vi "Christinas Flow Control Program.vi"() -> ()   [LabVIEW 2015]
uses:
  Alicat Device.lvclass
  Reusable/Session APIs/File Access/Config Data/Config Session.ctl
  Reusable/Session APIs/File Access/Config Data/Config Data.lvclass
  Reusable/Session APIs/Serial/Serial Session.lvclass
  <userlib>/_Session Fwk/Typedefs/Session Handle.ctl
  <userlib>/_Session Fwk/Session - Root.lvclass
  Reusable/Session Log/System Log.lvclass
  Reusable/Session Log/System Log.lvclass/System Log.ctl
  Reusable/Session APIs/File Access/Config Data/Config Data.lvclass/Config Data.ctl
  Reusable/Session APIs/Text Communication/Text Device Session.lvclass/Text Device Session.ctl
  Configurable Device/Configurable Device.lvclass/Configurable Device.ctl
  Alicat Device.lvclass/Alicat Device.ctl
  Data/Alicat Data.lvclass
  Reusable/Session APIs/Text Communication/Write hSysLog.vi
  Configurable Device/Write Handle.vi
  Accessors/Write ID.vi
  Accessors/Write Session Handle.vi
  Accessors/Read Type.vi
  Reusable/Session Log/Accessors/Write Main Path.vi
  Reusable/Session APIs/File Access/Config Data/Accessors/Write Cfg Path.vi
  Reusable/Data/Read measTime.vi
  Reusable/Data/Data.lvclass
panel:
  in  "Limonene SP":dbl
  in  "Nitrogen SP":dbl
  in  "Ozone SP":dbl
  out "error out":errorcluster
  out "Acquisition Time":timestamp format="%<%H:%M:%S%2u>T"
  out "Limonene":T1
  out "Nitrogen":T1
  out "Ozone":T1
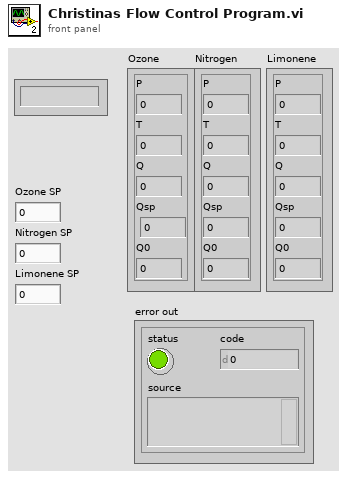
[diagram p1: front panel]
types:
  T1 = cluster{"P":dbl, "T":dbl, "Q":dbl, "Qsp":dbl, "Q0":dbl}
  T2 = typedef "Session - Root.lvclass/Session Handle.ctl" = refnum<data-value>
  T3 = typedef "Config Data.lvclass/Config Session.ctl" = refnum<data-value>
  T4 = cluster{"Accessors:Data[0]":sgl, "Accessors:Data[1]":sgl, "Accessors:Data[2]":sgl, "Accessors:Data[3]":sgl, "Accessors:Data[4]":sgl}
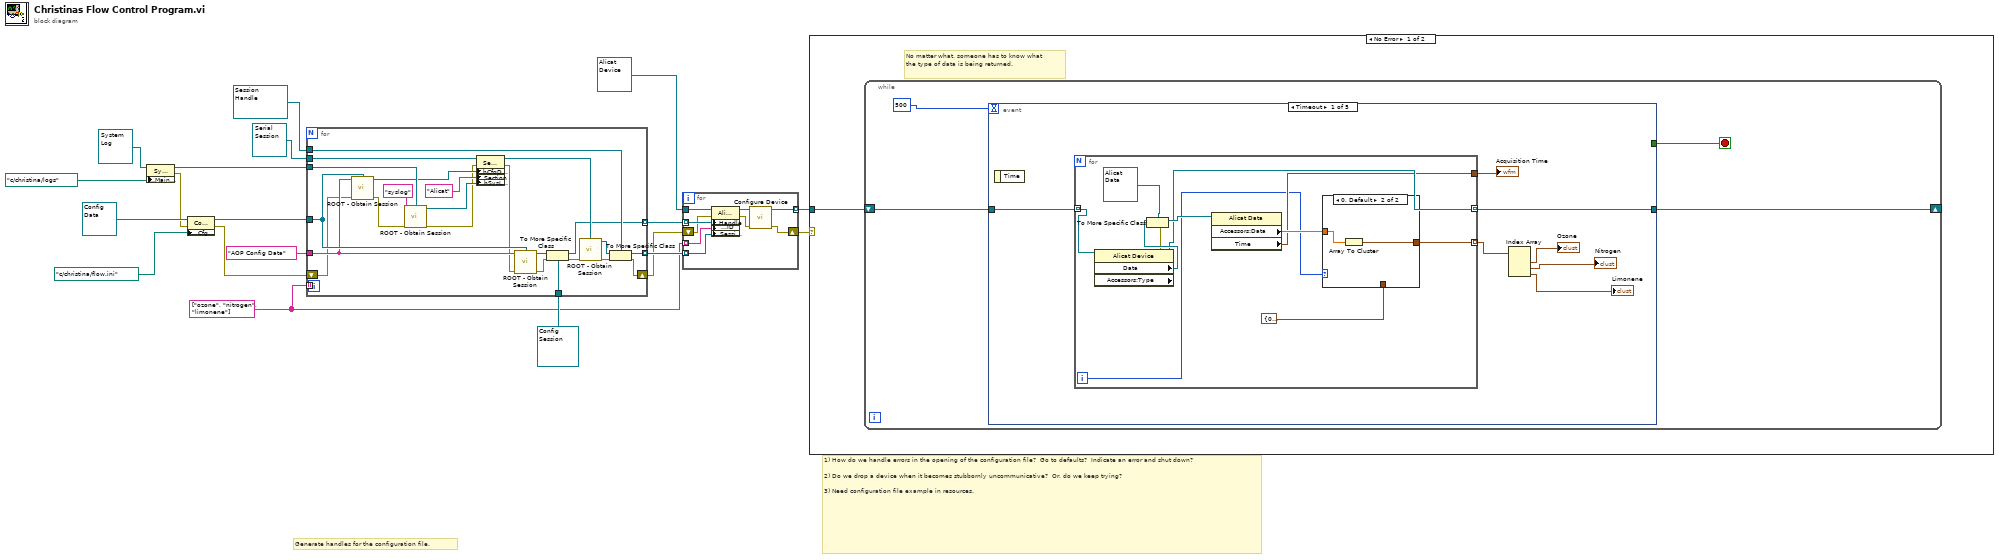
[diagram p0: block diagram]
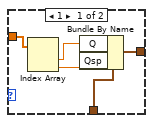
[diagram p2: hidden frame]
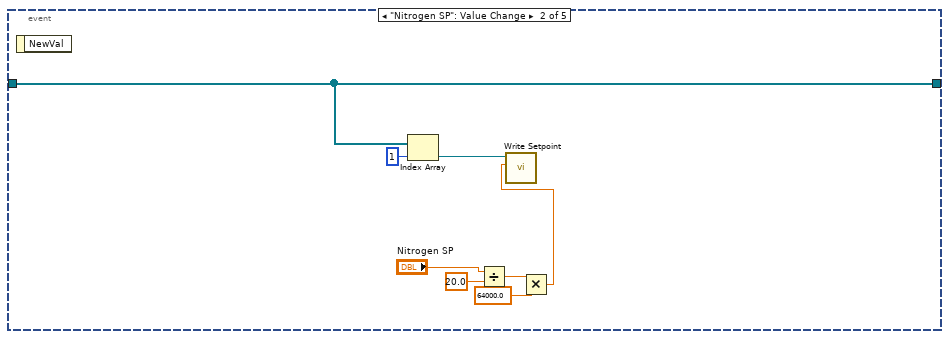
[diagram p3: hidden frame]
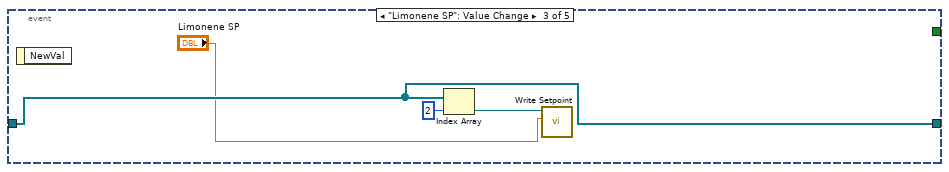
[diagram p4: hidden frame]
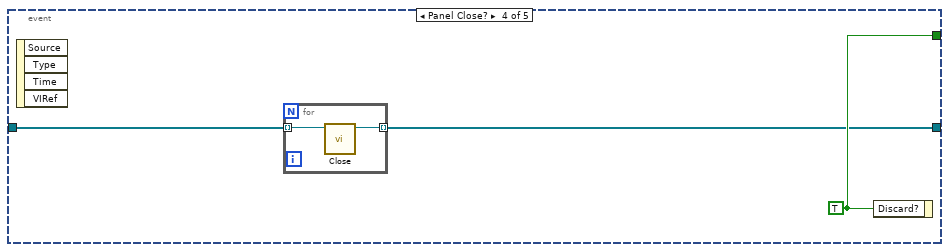
[diagram p5: hidden frame]
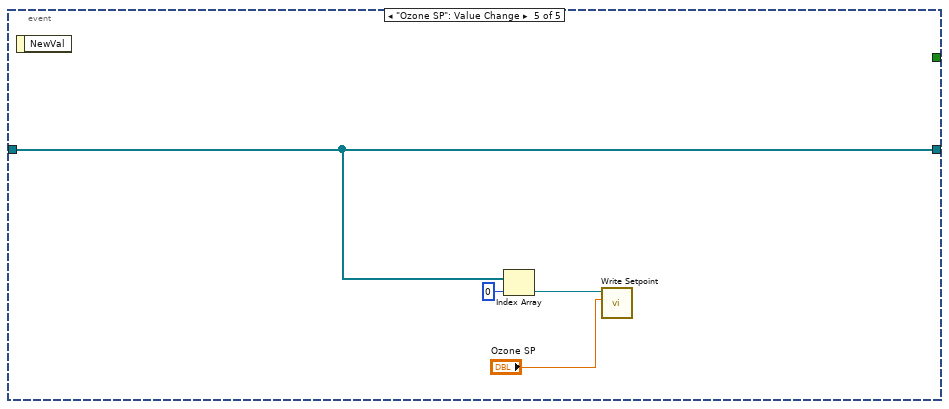
[diagram p6: hidden frame]
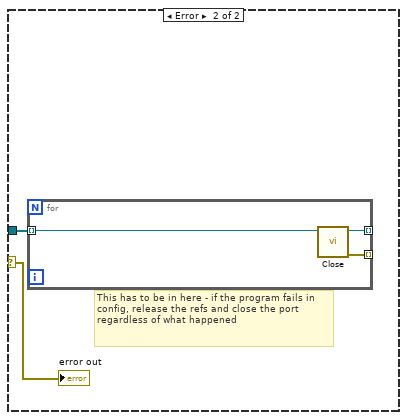
[diagram p7: hidden frame]
diagram:
  w2 = string[] ["ozone", "nitrogen", "limonene"] ("Array")
  # "1) How do we handle errors in the opening of the configuration file?  Go to defaults?  Indicate an error and shut down?\n\n2) Do we drop a device when it becomes stubbornly uncommunicative?  Or, do we keep trying?\n\n3) Need configuration file example in resources."
  # "Generate handles for the configuration file."
  n1 = property class="Sys Log"(reference=refnum<class "System Log.lvclass"> refnum ("Sys Log"), "Accessors:Main Path"=path "c:/christina/logs" ("Main Path")) -> (reference out=w9:refnum<class "System Log.lvclass">, error out=w4:errorcluster)  [unwired: 1 in]
  n2 = property class="Config Data"(reference=refnum<class "Config Data.lvclass"> refnum ("Config Data"), error in=w4, "Accessors:Cfg Path"=path "c:/christina/flow.ini" ("Path")) -> (reference out=w7:refnum<class "Config Data.lvclass">, error out=w3:errorcluster)
  n3 = for {
    tunnel: T3 refnum ("Session Handle") -> [w42]
    tunnel: [w28] -> w6 mode=indexing
    tunnel: "AOP Config Data" ("Session Name ()") -> [w26]
    tunnel: refnum<class "Serial Session.lvclass"> refnum ("Serial Session") -> [w40]
    tunnel: T2 refnum ("Session Handle") -> [w36]
    tunnel: [w35] -> w12 mode=indexing
    tunnel: w9 -> [w34]
    tunnel: w2 -> [_] mode=indexing
    tunnel: w7 -> [w27]
    shift-right: [w24] -> w1
    shift-left: w3 -> [w23]
    n4 = call <userlib>:"ROOT - Obtain Session.vi"("Session Name ()"=w26, "OBJ - Session"=w27, "error in (no error)"=w23) -> ("Session Handle"=w25:T2, "error out"=w22:errorcluster)  [unwired: 10 in, 1 out]
    n5 = call <userlib>:"ROOT - Obtain Session.vi"("Session Name ()"="syslog", "OBJ - Session"=w34, "error in (no error)"=w22) -> ("Session Handle"=w32:T2, "error out"=w21:errorcluster)  [unwired: 10 in, 1 out]
    n6 = property class="Serial Session"(reference=w40, error in=w21, "Accessors:hCfgData"=w25, "Accessors:Section"="Alicat" ("Section"), "Accessors:hSysLog"=w32) -> (reference out=w39:refnum<class "Serial Session.lvclass">, error out=w20:errorcluster)
    n7 = call <userlib>:"ROOT - Obtain Session.vi"("Session Name ()"=w26, "OBJ - Session"=w27, "error in (no error)"=w20) -> ("Session Handle"=w31:T2, "error out"=w41:errorcluster)  [unwired: 10 in, 1 out]
    n8 = To More Specific Class(target class=w42, reference=w31, error in=w41) -> (specific class reference=w28:T3, error out=w30:errorcluster)
    n9 = call <userlib>:"ROOT - Obtain Session.vi"("OBJ - Session"=w39, "error in (no error)"=w30) -> ("Session Handle"=w37:T2, "error out"=w29:errorcluster)  [unwired: 11 in, 1 out]
    n10 = To More Specific Class(target class=w36, reference=w37, error in=w29) -> (specific class reference=w35:T2, error out=w24:errorcluster)
  }
  n11 = for {
    tunnel: w2 -> [w50] mode=indexing
    tunnel: [w46] -> w18 mode=indexing
    tunnel: refnum<class "Alicat Device.lvclass"> refnum ("Alicat Device in") -> [w51]
    tunnel: w6 -> [w49] mode=indexing
    tunnel: w12 -> [w44] mode=indexing
    shift-right: [w45] -> w19
    shift-left: w1 -> [w43]
    n12 = property class="Alicat Device"(reference=w51, error in=w43, "Accessors:Handle"=w49, "Accessors:ID"=w50, "Accessors:Session Handle"=w44) -> (reference out=w47:refnum<class "Alicat Device.lvclass">, error out=w48:errorcluster)
    n13 = call-dynamic "Configure Device.vi"("error in"=w48, "Alicat Device in"=w47) -> ("error out"=w45:errorcluster, "Alicat Device out"=w46:refnum<class "Alicat Device.lvclass">)  [unwired: 8 in]
  }
  n14 = case shown="No Error" w19 {
    selector: w19 -> [_ w103]
    tunnel: w18 -> [w52 w104]
    frame No Error {
      # "No matter what, someone has to know what the type of data is being returned."
      n15 = while {
        shift-right: [w55] -> _
        shift-left: w52 -> [w56]
        stop <- w53 stop-if-true
        n16 = event shown="[0] Timeout" {
          selector: _ -> [_ _ _ _ _]
          dyn-events: _ -> [_ _ _ _ _]
          timeout: 500 -> [_ _ _ _ _]
          tunnel: w56 -> [w63 w89 w91 w95 w100]
          tunnel: [w62 w89 w91 w94 w100] -> w55
          tunnel: [_ _ _ w96 _] -> w53
          event Timeout {
            n17 = event-data() -> ()  [unwired: 1 in, 1 out]
            n18 = for {
              tunnel: [w71] -> w62 mode=indexing
              tunnel: w63 -> [w73] mode=indexing
              tunnel: [w67] -> w61 mode=indexing
              tunnel: [w66] -> w57
              i -> [w64]
              n19 = property class="Alicat Device" props=["Data", "Accessors:Type"](reference=w73) -> (reference out=w71:refnum<class "Alicat Device.lvclass">, error out=w70:errorcluster, "Data"=w72:refnum<class "Data.lvclass">)  [unwired: 1 in, 1 out]
              n20 = To More Specific Class(target class=refnum<class "Alicat Data.lvclass"> refnum ("Alicat Data"), reference=w72, error in=w70) -> (specific class reference=w74:refnum<class "Alicat Data.lvclass">)  [unwired: 1 out]
              n21 = property class="Alicat Data"(reference=w74) -> ("Accessors:Data"=w69:sgl[], "Time"=w66:timestamp)  [unwired: 1 in, 2 out]
              n22 = case shown="0, Default" w64 {
                tunnel: w69 -> [w79 w81]
                tunnel: T1 {"P"=0.0, "T"=0.0, "Q"=0.0, "Qsp"=0.0, "Q0"=0.0} ("FC 1") -> [w77 _]
                tunnel: [w76 w80] -> w67
                frame 1 {
                  n23 = Index Array(array=w79) -> (element #1=w78:sgl, element #2=w75:sgl)  [unwired: 2 in]
                  n24 = Bundle By Name(cluster=w77, "Q"=w78, "Qsp"=w75) -> (w76:T1)
                }
                frame 0, Default {
                  n25 = Array To Cluster(array=w81) -> (cluster=w80:T4)
                }
              }
            }
            "Acquisition Time" <- w57
            n26 = Index Array(array=w61) -> (element #1=→"Ozone":T1, element #2=→"Nitrogen":T1, element #3=→"Limonene":T1)  [unwired: 3 in]
          }
          event "Nitrogen SP": Value Change {
            n27 = event-data() -> ()  [unwired: 1 in, 1 out]
            n28 = Index Array(array=w89, index=1) -> (element=w87:refnum<class "Alicat Device.lvclass">)
            n29 = Divide(x="Nitrogen SP", y=20.0) -> (x/y=w84:dbl)
            n30 = Multiply(x=w84, y=64000.0) -> (x*y=w82:dbl)
            n31 = call "Write Setpoint.vi"("Setpoint"=w82, "Alicat Device in"=w87) -> ()  [unwired: 7 in, 3 out]
          }
          event "Limonene SP": Value Change {
            n32 = event-data() -> ()  [unwired: 1 in, 1 out]
            n33 = Index Array(array=w91, index=2) -> (element=w92:refnum<class "Alicat Device.lvclass">)
            n34 = call "Write Setpoint.vi"("Setpoint"="Limonene SP", "Alicat Device in"=w92) -> ()  [unwired: 7 in, 3 out]
          }
          event Panel Close? {
            w96 = TRUE ("Discard?")
            n35 = event-data() -> ()  [unwired: 1 in, 4 out]
            n36 = for {
              tunnel: [w97] -> w94 mode=indexing
              tunnel: w95 -> [w98] mode=indexing
              n37 = call-dynamic "Close.vi"("Cfg Dev in"=w98) -> ("Cfg Dev out"=w97:refnum<class "Alicat Device.lvclass">)  [unwired: 9 in, 1 out]
            }
            n38 = event-data("Discard?"=w96) -> ()  [unwired: 1 in, 1 out]
          }
          event "Ozone SP": Value Change {
            n39 = event-data() -> ()  [unwired: 1 in, 1 out]
            n40 = Index Array(array=w100, index=0) -> (element=w101:refnum<class "Alicat Device.lvclass">)
            n41 = call "Write Setpoint.vi"("Setpoint"="Ozone SP", "Alicat Device in"=w101) -> ()  [unwired: 7 in, 3 out]
          }
        }
      }
    }
    frame Error {
      # "This has to be in here - if the program fails in config, release the refs and close the port regardless of what happened"
      n42 = for {
        tunnel: [w106] -> _ mode=indexing
        tunnel: [w105] -> _ mode=indexing
        tunnel: w104 -> [w107] mode=indexing
        n43 = call-dynamic "Close.vi"("Cfg Dev in"=w107) -> ("error out"=w105:errorcluster, "Cfg Dev out"=w106:refnum<class "Alicat Device.lvclass">)  [unwired: 9 in]
      }
      "error out" <- w103
    }
  }
